vi "MagnaDC Output Voltage.vi"() -> ()   [LabVIEW 2022 SP3]
doc: "Simple example how to control power supplu output using voltage and current levels."
uses:
  <vilib>/Utility/error.llb/DialogType.ctl
  Magna sub vis/MagnaDC.lvlib
panel:
  out "OCP Tripped":bool
  out "OVP Tripped":bool
  out "Current (A)":dbl=0.2
  out "Voltage (V)":dbl=203.0
  in  "Stop":bool
  in  "Output":bool=TRUE
  in  "OCP (A)":dbl=6.0 format="%.2f"
  in  "OVP (V)":dbl=280.0 format="%.2f"
  in  "Current Limit (A)":dbl=5.0 format="%.2f"
  in  "Voltage Limit (V)":dbl=203.0 format="%.2f"
  out "error out":errorcluster
  in  "error in (no error)":errorcluster
  in  "VISA resource name":refnum<visa-resource-name>="TCPIP0::131.227.181.163::50505::SOCKET"
  # "(c) 2004 - 2018 Magna-Power Electronics Inc.  ALL RIGHTS RESERVED."
  # "Enabled"
  # "Disabled"
  # "Instrument Settings"
  # "Output Values"
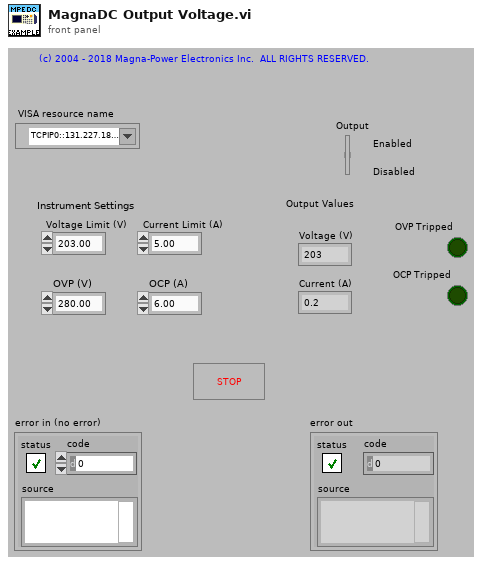
[diagram p1: front panel]
types:
  T1 = enum8{"Enabled", "Disabled", "Disabled and Grayed Out"}
  T2 = typedef "DialogType.ctl" = u16
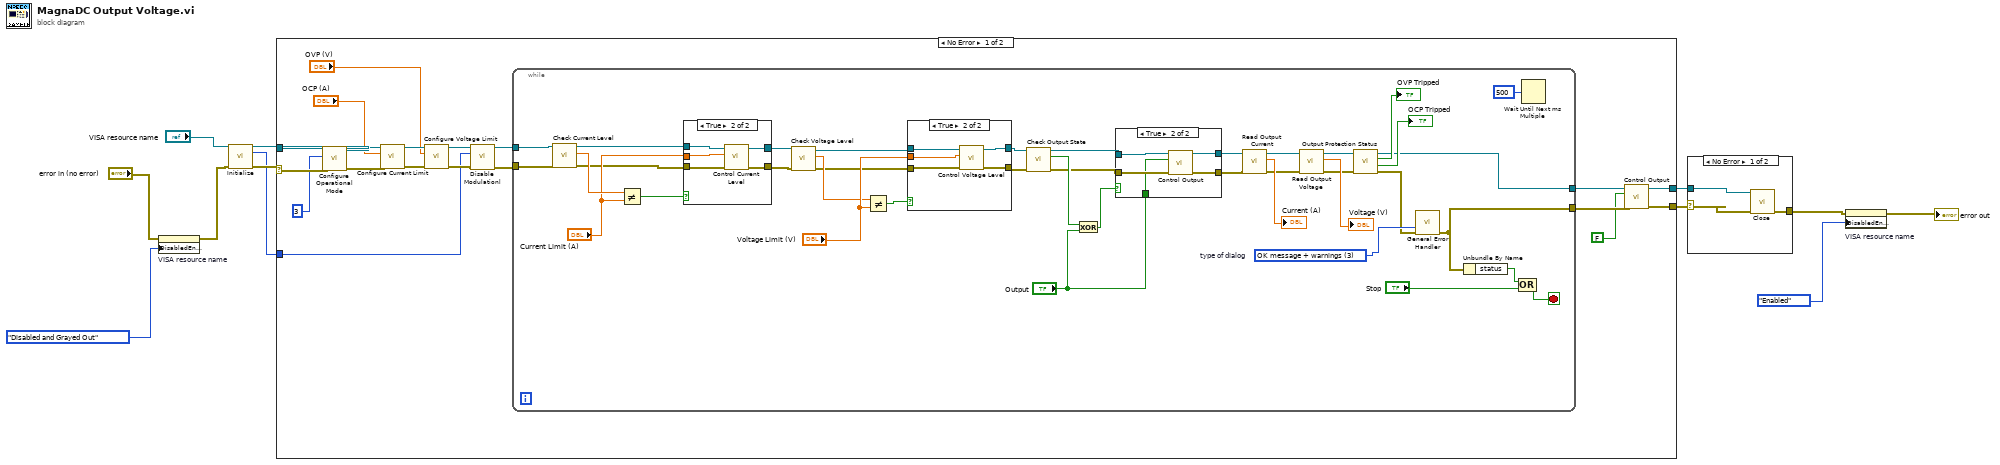
[diagram p0: block diagram]
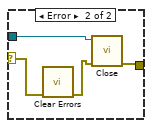
[diagram p2: hidden frame]
diagram:
  n1 = property on="VISA resource name" class="VISAName"(error in="error in (no error)", "DisabledEnum"=T1."Disabled and Grayed Out" ("Disabled")) -> (error out=w3:errorcluster)  [unwired: 1 in, 1 out]
  n2 = call "Initialize.vi"("VISA resource name"="VISA resource name", "error in (no error)"=w3) -> ("VISA resource name out"=w10:refnum<visa-resource-name>, "Modulation Available"=w1:u32, "error out"=w11:errorcluster)  [unwired: 10 in, 1 out]
  n3 = case shown="No Error" w11 {
    selector: w11 -> [w30 w93]
    tunnel: w10 -> [w31 w92]
    tunnel: [w27 w93] -> w8
    tunnel: [w28 w92] -> w7
    tunnel: w1 -> [w13 _]
    frame No Error {
      n4 = call "Configure Operational Mode.vi"("error in (no error)"=w30, "Operational Mode"=u32 3, "VISA resource name"=w31) -> ("error out"=w21:errorcluster, "VISA resource name out"=w23:refnum<visa-resource-name>)  [unwired: 7 in]
      n5 = call "Configure Current Limit.vi"("error in (no error)"=w21, "Current Limit (0.0 A)"="OCP (A)", "VISA resource name"=w23) -> ("error out"=w20:errorcluster, "VISA resource name out"=w22:refnum<visa-resource-name>)  [unwired: 7 in]
      n6 = call "Configure Voltage Limit.vi"("error in (no error)"=w20, "Voltage Limit (0.0 V)"="OVP (V)", "VISA resource name"=w22) -> ("error out"=w17:errorcluster, "VISA resource name out"=w16:refnum<visa-resource-name>)  [unwired: 7 in]
      n7 = call "Disable Modulationl.vi"("VISA resource name"=w16, "Modulation"=w13, "error in (no error)"=w17) -> ("VISA resource name out"=w15:refnum<visa-resource-name>, "error out"=w14:errorcluster)  [unwired: 11 in]
      n8 = while {
        tunnel: [w56] -> w25
        tunnel: [w55] -> w26
        tunnel: w15 -> [w33]
        tunnel: w14 -> [w32]
        stop <- w69 stop-if-true
        w58 = T2 3 items=["no dialog", "OK message", "continue or stop message", "OK message + warnings", "continue/stop + warnings"]  # type of dialog
        n9 = call "Check Current Level.vi"("error in (no error)"=w32, "VISA resource name"=w33) -> ("error out"=w37:errorcluster, "Current Level (A)"=w40:dbl, "VISA resource name out"=w36:refnum<visa-resource-name>)  [unwired: 7 in]
        n10 = Not Equal?(x=w40, y="Current Limit (A)") -> (x != y?=w38:bool)
        n11 = case shown="True" w38 {
          tunnel: w37 -> [w78 w84]
          tunnel: w36 -> [w79 w83]
          tunnel: [w79 w82] -> w43
          tunnel: [w78 w81] -> w44
          tunnel: "Current Limit (A)" -> [_ w80]
          frame False {
          }
          frame True {
            n12 = call "Control Current Level.vi"("error in (no error)"=w84, "Current Level (0.0 A)"=w80, "VISA resource name"=w83) -> ("error out"=w81:errorcluster, "VISA resource name out"=w82:refnum<visa-resource-name>)  [unwired: 7 in]
          }
        }
        n13 = call "Check Voltage Level.vi"("error in (no error)"=w44, "VISA resource name"=w43) -> ("error out"=w42:errorcluster, "Voltage Level (V)"=w46:dbl, "VISA resource name out"=w41:refnum<visa-resource-name>)  [unwired: 7 in]
        n14 = Not Equal?(x=w46, y="Voltage Limit (V)") -> (x != y?=w45:bool)
        n15 = case shown="True" w45 {
          tunnel: w41 -> [w72 w77]
          tunnel: w42 -> [w71 w76]
          tunnel: [w72 w75] -> w35
          tunnel: [w71 w74] -> w34
          tunnel: "Voltage Limit (V)" -> [_ w73]
          frame False {
          }
          frame True {
            n16 = call "Control Voltage Level.vi"("error in (no error)"=w76, "Voltage Level (0.0 V)"=w73, "VISA resource name"=w77) -> ("error out"=w74:errorcluster, "VISA resource name out"=w75:refnum<visa-resource-name>)  [unwired: 7 in]
          }
        }
        n17 = call "Check Output State.vi"("error in (no error)"=w34, "VISA resource name"=w35) -> ("error out"=w51:errorcluster, "Output"=w54:bool, "VISA resource name out"=w52:refnum<visa-resource-name>)  [unwired: 7 in]
        n18 = Exclusive Or(1:"Output", 2:w54) -> (0:w53:bool)
        n19 = case shown="True" w53 {
          tunnel: w52 -> [w86 w91]
          tunnel: w51 -> [w85 w90]
          tunnel: [w86 w89] -> w50
          tunnel: [w85 w88] -> w49
          tunnel: "Output" -> [_ w87]
          frame False {
          }
          frame True {
            n20 = call "Control Output.vi"("error in (no error)"=w90, "Enable Output (T: Enable)"=w87, "VISA resource name"=w91) -> ("error out"=w88:errorcluster, "VISA resource name out"=w89:refnum<visa-resource-name>)  [unwired: 7 in]
          }
        }
        n21 = call "Read Output Current.vi"("error in (no error)"=w49, "VISA resource name"=w50) -> ("error out"=w65:errorcluster, "Actual Current Level (A)"=→"Current (A)":dbl, "VISA resource name out"=w66:refnum<visa-resource-name>)  [unwired: 6 in]
        n22 = call "Read Output Voltage.vi"("error in (no error)"=w65, "VISA resource name"=w66) -> ("error out"=w60:errorcluster, "Actual Voltage Level (V)"=→"Voltage (V)":dbl, "VISA resource name out"=w61:refnum<visa-resource-name>)  [unwired: 7 in]
        n23 = call "Output Protection Status.vi"("error in (no error)"=w60, "VISA resource name"=w61) -> ("error out"=w57:errorcluster, "OCP Tripped"=→"OCP Tripped":bool, "OVP Tripped"=→"OVP Tripped":bool, "VISA resource name out"=w55:refnum<visa-resource-name>)  [unwired: 6 in]
        n24 = call <vilib>:"General Error Handler.vi"("type of dialog (OK msg:1)"=w58, "error in (no error)"=w57) -> ("error out"=w56:errorcluster)  [unwired: 9 in, 4 out]
        n25 = Unbundle By Name(w56) -> ("status"=w59:bool)
        n26 = Compound Arithmetic op=OR(w59, "Stop") -> (w69:bool)
        n27 = Wait Until Next ms Multiple(millisecond multiple=u32 500) -> ()  [unwired: 1 out]
      }
      n28 = call "Control Output.vi"("error in (no error)"=w25, "Enable Output (T: Enable)"=FALSE, "VISA resource name"=w26) -> ("error out"=w27:errorcluster, "VISA resource name out"=w28:refnum<visa-resource-name>)  [unwired: 7 in]
    }
    frame Error {
    }
  }
  n29 = case shown="No Error" w8 {
    selector: w8 -> [w96 w100]
    tunnel: [w94 w98] -> w6
    tunnel: w7 -> [w95 w97]
    frame No Error {
      n30 = call "Close.vi"("error in (no error)"=w96, "VISA resource name"=w95) -> ("error out"=w94:errorcluster)  [unwired: 9 in]
    }
    frame Error {
      n31 = call <vilib>:"Clear Errors.vi"("error in (no error)"=w100) -> ("error out"=w99:errorcluster)  [unwired: 5 in, 1 out]
      n32 = call "Close.vi"("error in (no error)"=w99, "VISA resource name"=w97) -> ("error out"=w98:errorcluster)  [unwired: 9 in]
    }
  }
  n33 = property on="VISA resource name" class="VISAName"(error in=w6, "DisabledEnum"=T1."Enabled" ("Disabled")) -> (error out=→"error out":errorcluster)  [unwired: 1 in, 1 out]
